vi "RS-xxx Factory.vi"(8 "error in (no error)":errorcluster, 10 "settings":T1) -> (0 "error out":errorcluster, 3 "protocol out":refnum<class "Protocol Parent.lvclass">)   [LabVIEW 2020, in "Instrument Addon Scripting API.lvlib"]
doc: "Instantiate a new RS-xxx Protocol object using the provided RS-xxx Port settings."
uses:
  Instrument Addon Scripting API.lvlib
  Libraries Directory/Protocols.lvlibp/RS-xxx/RS-xxx Settings.ctl
  Libraries Directory/Protocols.lvlibp/Protocol Parent/Protocol Parent.lvclass
  Libraries Directory/Protocols.lvlibp/RS-xxx/RS-xxx.lvclass
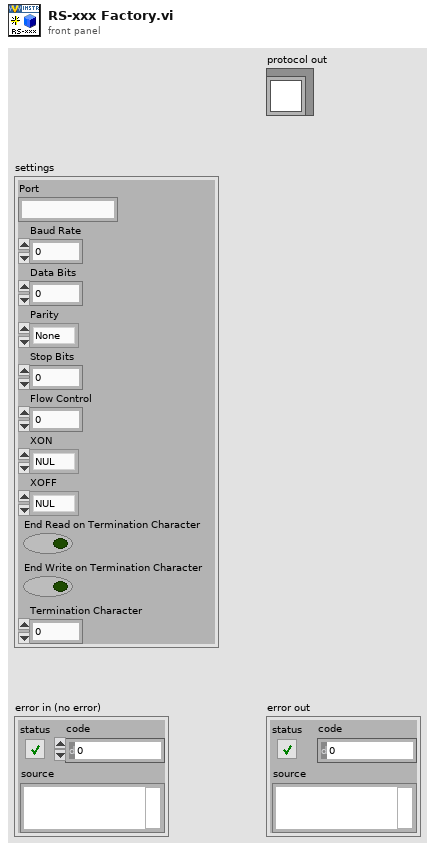
[diagram p1: front panel]
types:
  T1 = typedef "Protocols.lvlibp/RS-xxx.lvclass/RS-xxx Settings.ctl" = cluster{"Port":string, "Baud Rate":u32, "Data Bits":u16, "Parity":enum16{"None", "Odd", "Even", "Mark", "Space"}, "Stop Bits":u16, "Flow Control":u16, "XON":enum16{"NUL", "SOH", "STX", "ETX", "EOT", "ENQ", "ACK", "BEL", "BS", "HT", "LF", "VT", "FF", "CR", "SO", "SI", "DLE", "DC1", "DC2", "DC3", "DC4", "NAK", "SYN", "ETB", "CAN", "EM", "SUB", "ESC", "FS", "GS", "RS", "US", "SP", "!", "\"", "#", "$", "%", "&", "'", "(", ")", "*", "+", ",", "- (-)", ".", "/", "0", "1", "2", "3", "4", "5", "6", "7", "8", "9", ":", ";", "<", "=", ">", "?", "@", "A", "B", "C", "D", "E", "F", "G", "H", "I", "J", "K", "L", "M", "N", "O", "P", "Q", "R", "S", "T", "U", "V", "W", "X", "Y", "Z", "[", "\\", "]", "^", "_", "`", "a", "b", "c", "d", "e", "f", "g", "h", "i", "j", "k", "l", "m", "n", "o", "p", "q", "r", "s", "t", "u", "v", "w", "x", "y", "z", "{", "|", "}", "~"}, "XOFF":enum16{"NUL", "SOH", "STX", "ETX", "EOT", "ENQ", "ACK", "BEL", "BS", "HT", "LF", "VT", "FF", "CR", "SO", "SI", "DLE", "DC1", "DC2", "DC3", "DC4", "NAK", "SYN", "ETB", "CAN", "EM", "SUB", "ESC", "FS", "GS", "RS", "US", "SP", "!", "\"", "#", "$", "%", "&", "'", "(", ")", "*", "+", ",", "- (-)", ".", "/", "0", "1", "2", "3", "4", "5", "6", "7", "8", "9", ":", ";", "<", "=", ">", "?", "@", "A", "B", "C", "D", "E", "F", "G", "H", "I", "J", "K", "L", "M", "N", "O", "P", "Q", "R", "S", "T", "U", "V", "W", "X", "Y", "Z", "[", "\\", "]", "^", "_", "`", "a", "b", "c", "d", "e", "f", "g", "h", "i", "j", "k", "l", "m", "n", "o", "p", "q", "r", "s", "t", "u", "v", "w", "x", "y", "z", "{", "|", "}", "~"}, "End Read on Termination Character":bool, "End Write on Termination Character":bool, "Termination Character":u8}
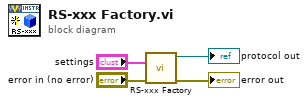
[diagram p0: block diagram]
diagram:
  n1 = call "RS-xxx Factory.vi"("error in (no error)"="error in (no error)", "RS-xxx settings"="settings") -> ("error out"=→"error out":errorcluster, "protocol out"=→"protocol out":refnum<class "Protocol Parent.lvclass">)  [unwired: 8 in]
